vi "get_status_modelocked.vi"(8 "error in (no error)":errorcluster, 11 "LightSourceAN191011Chameleon in":refnum<class "LightSourceAN191011Chameleon.lvclass">) -> (0 "error out":errorcluster, 1 "Emission":bool, 2 "Pulsing":bool, 3 "LightSourceAN191011Chameleon out":refnum<class "LightSourceAN191011Chameleon.lvclass">)   [LabVIEW 2010, in "LightSourceAN191011Chameleon.lvclass"]
uses:
  LightSourceAN191011Chameleon.lvclass
  LightSourceAN191011Chameleon.lvclass/LightSourceAN191011Chameleon.ctl
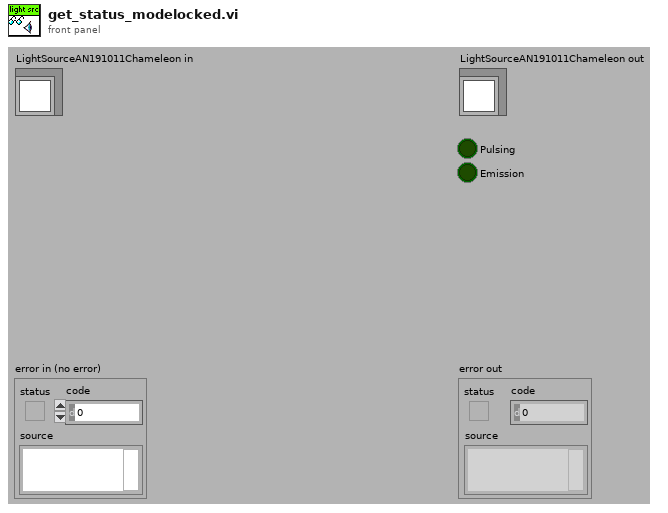
[diagram p1: front panel]
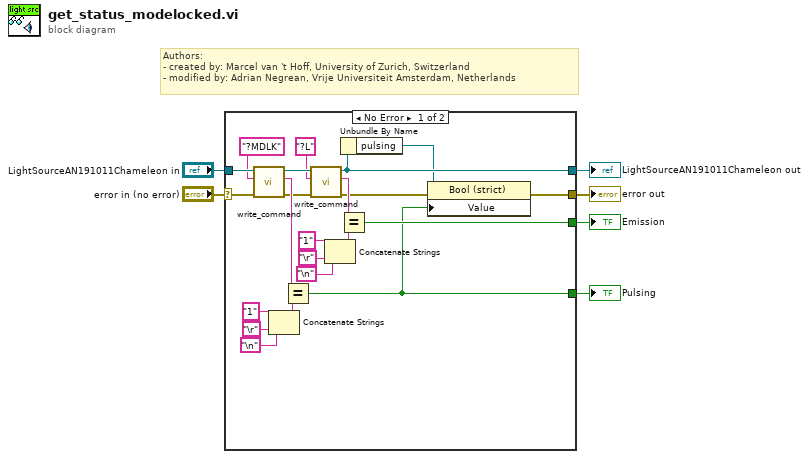
[diagram p0: block diagram]
diagram:
  # "Authors: \n- created by: Marcel van 't Hoff, University of Zurich, Switzerland\n- modified by: Adrian Negrean, Vrije Universiteit Amsterdam, Netherlands"
  n1 = case shown="No Error" "error in (no error)" {
    selector: "error in (no error)" -> [w27 w30]
    tunnel: [w8 w30] -> w5
    tunnel: [w11 w29] -> w3
    tunnel: "LightSourceAN191011Chameleon in" -> [w28 w29]
    tunnel: [w7 _] -> w2
    tunnel: [w12 _] -> w1
    frame No Error {
      n2 = call-dynamic "write_command.vi"("error in (no error)"=w27, "string to write"="?MDLK", "LightSourceAN191011Chameleon in"=w28) -> ("error out"=w19:errorcluster, "read string"=w21:string, "LightSourceAN191011Chameleon out"=w20:refnum<class "LightSourceAN191011Chameleon.lvclass">)  [unwired: 6 in]
      n3 = Concatenate Strings("1" ("string"), "\r", "\n") -> (w22:string)
      n4 = Equal?(x=w21, y=w22) -> (x = y?=w7:bool)
      n5 = call-dynamic "write_command.vi"("error in (no error)"=w19, "string to write"="?L", "LightSourceAN191011Chameleon in"=w20) -> ("error out"=w9:errorcluster, "read string"=w13:string, "LightSourceAN191011Chameleon out"=w11:refnum<class "LightSourceAN191011Chameleon.lvclass">)  [unwired: 6 in]
      n6 = Concatenate Strings("1" ("string"), "\r", "\n") -> (w14:string)
      n7 = Equal?(x=w13, y=w14) -> (x = y?=w12:bool)
      n8 = Unbundle By Name(w11) -> ("pulsing"=w10:refnum<vi>)
      n9 = property class="Bool (strict)"(reference=w10, error in=w9, "Value"=w7) -> (error out=w8:errorcluster)  [unwired: 1 out]
    }
    frame Error {
    }
  }
  "error out" <- w5
  "LightSourceAN191011Chameleon out" <- w3
  "Emission" <- w1
  "Pulsing" <- w2
